vi "Jacobian Demo.vi"() -> ()   [LabVIEW 2017, in "NI_Kinematics.lvlib"]
uses:
  <vilib>/robotics/Kinematics/NI_Kinematics.lvlib
  <vilib>/Analysis/Matrix/Datatypes/RealMatrix.ctl
  <vilib>/Analysis/Matrix/NI_Matrix.lvlib
panel:
  out "World Frame Jacobian":T1
  out "End Effector Time (ms)":u32
  out "End Effector Jacobian":T1
  out "World Time (ms)":u32
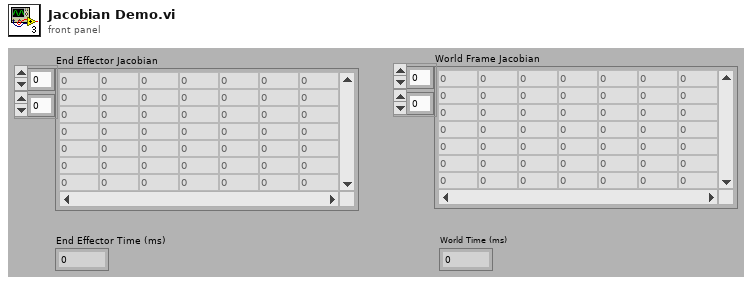
[diagram p1: front panel]
types:
  T1 = typedef "NI_Matrix.lvlib/RealMatrix.ctl" = dbl[][]
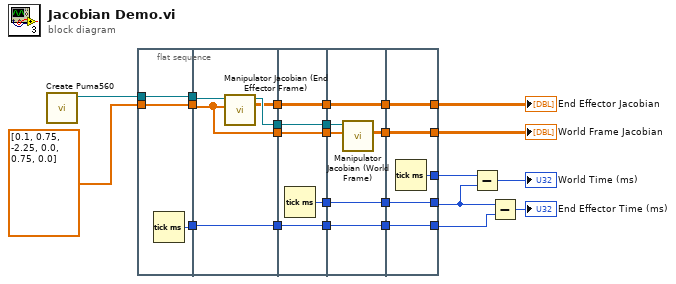
[diagram p0: block diagram]
diagram:
  n1 = call <vilib>:"Create Puma560.vi"() -> ("Puma560 Robot"=w19:refnum<class "NI_Robotics_Serial Robot Arm.lvclass">)  [unwired: 1 in, 10 out]
  n2 = flat-sequence {
    tunnel: w19 -> [w28]
    tunnel: [w28] -> w25
    tunnel: [w27] -> w24
    tunnel: dbl[] [0.1, 0.75, -2.25, 0.0, 0.75, 0.0] ("positions") -> [w26]
    tunnel: [w26] -> w23
    tunnel: w25 -> [w32]
    tunnel: w24 -> [w33]
    tunnel: [w33] -> w22
    tunnel: w23 -> [w31]
    tunnel: [w31] -> w10
    tunnel: [w30] -> w8
    tunnel: [w29] -> w7
    tunnel: w22 -> [w38]
    tunnel: [w38] -> w18
    tunnel: [w37] -> w17
    tunnel: [w36] -> w16
    tunnel: [w35] -> w11
    tunnel: w10 -> [w35]
    tunnel: [w34] -> w9
    tunnel: w8 -> [w34]
    tunnel: w7 -> [w36]
    tunnel: w18 -> [w44]
    tunnel: w17 -> [w43]
    tunnel: w16 -> [w42]
    tunnel: [w44] -> w15
    tunnel: [w43] -> w14
    tunnel: [w42] -> w13
    tunnel: w11 -> [w41]
    tunnel: w9 -> [w40]
    tunnel: [w39] -> w4
    tunnel: [w47] -> w20
    tunnel: [w48] -> w5
    tunnel: [w49] -> w21
    tunnel: w15 -> [w49]
    tunnel: w14 -> [w48]
    tunnel: w13 -> [w47]
    tunnel: [w46] -> w6
    tunnel: [w45] -> w3
    tunnel: w4 -> [w45]
    frame #0 {
      n3 = Tick Count (ms)() -> (millisecond timer value=w27:u32)
    }
    frame #1 {
      n4 = call <vilib>:"Manipulator Jacobian (End Effector Frame).vi"("joint positions"=w31, "serial arm in"=w32) -> ("jacobian"=w29:T1, "serial arm out"=w30:refnum<class "NI_Robotics_Serial Robot Arm.lvclass">)  [unwired: 6 in, 2 out]
    }
    frame #2 {
      n5 = Tick Count (ms)() -> (millisecond timer value=w37:u32)
    }
    frame #3 {
      n6 = call <vilib>:"Manipulator Jacobian (World Frame).vi"("joint positions"=w41, "serial arm in"=w40) -> ("jacobian"=w39:T1)  [unwired: 6 in, 3 out]
    }
    frame #4 {
      n7 = Tick Count (ms)() -> (millisecond timer value=w46:u32)
    }
  }
  n8 = Subtract(x=w6, y=w5) -> (x-y=→"World Time (ms)":u32)
  n9 = Subtract(x=w5, y=w21) -> (x-y=→"End Effector Time (ms)":u32)
  "End Effector Jacobian" <- w20
  "World Frame Jacobian" <- w3
